vi "ADCP_Processed_Bytes_To_Data_Packet.vi"(8 "error in (no error)":errorcluster, 9 "Processed Packet":u8[](array[numeric])=[0, 0, 0, 0, 0, 0, 0, 0, 0], 10 "Data Packet In":T2, 11 "ADCP in":refnum<class "ADCP.lvclass">) -> (0 "error out":errorcluster, 2 "Data Packet Out":T2, 3 "ADCP out":refnum<class "ADCP.lvclass">)   [LabVIEW 2017, in "ADCP.lvclass"]
uses:
  ADCP.lvclass
  ADCP_Data_Packet_Transmit_Mode.ctl
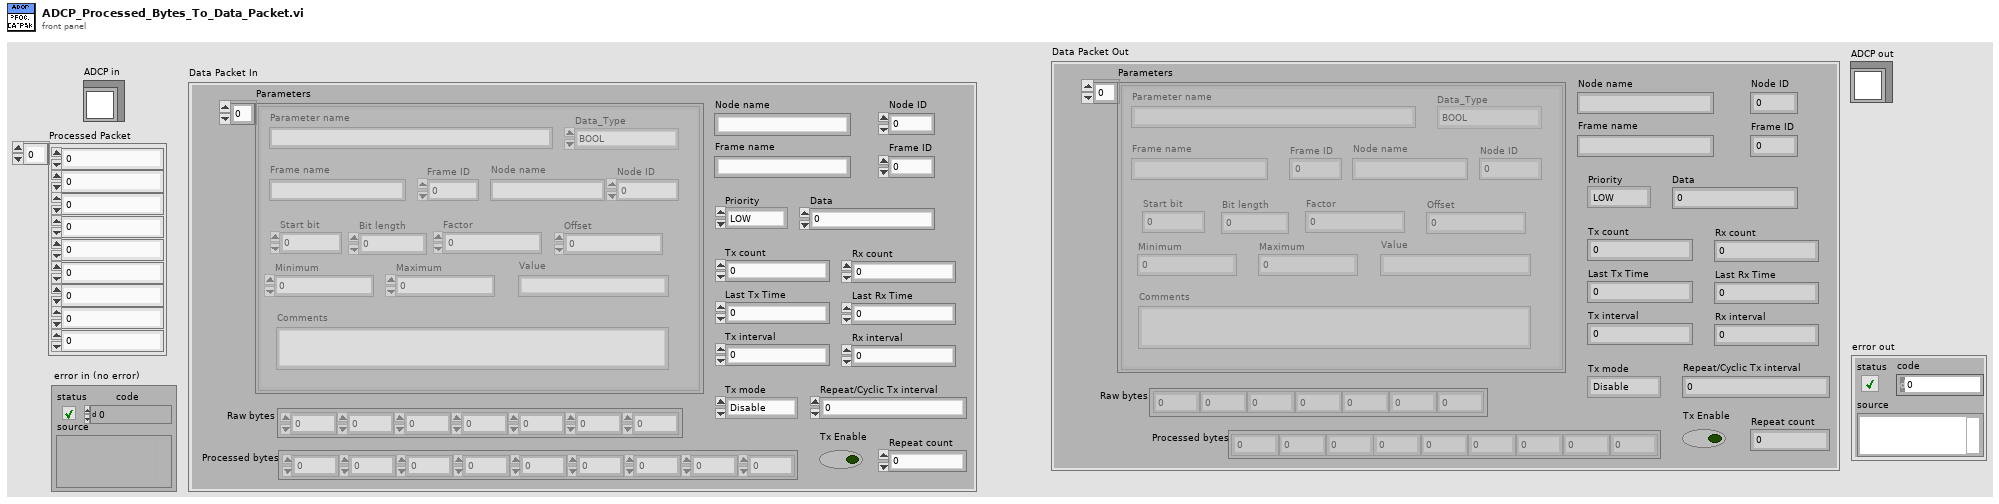
[diagram p1: front panel]
types:
  T1 = typedef "ADCP.lvclass/ADCP_Data_Packet_Transmit_Mode.ctl" = enum16{"Disable", "Single", "Cyclic", "Repeat"}
  T2 = cluster{"Parameters":cluster{"Parameter name":string, "Node name":string, "Node ID":u8, "Frame name":string, "Frame ID":u8, "Start bit":u32, "Bit length":u32, "Factor":dbl, "Offset":dbl, "Minimum":dbl, "Maximum":dbl, "Value":string, "Comments":string, "Data_Type":enum16{"BOOL", "UNSIGNED", "SIGNED", "FLOAT32", "ENUM"}}[], "Priority":enum16{"LOW", "HIGH"}, "Node name":string, "Node ID":u8, "Frame name":string, "Frame ID":u8, "Data":u32, "Raw bytes":u8[], "Processed bytes":u8[], "Tx count":i32, "Last Tx Time":u32, "Tx interval":u32, "Rx count":i32, "Last Rx Time":u32, "Rx interval":u32, "Tx Enable":bool, "Tx mode":T1, "Repeat/Cyclic Tx interval":u32, "Repeat count":u16}
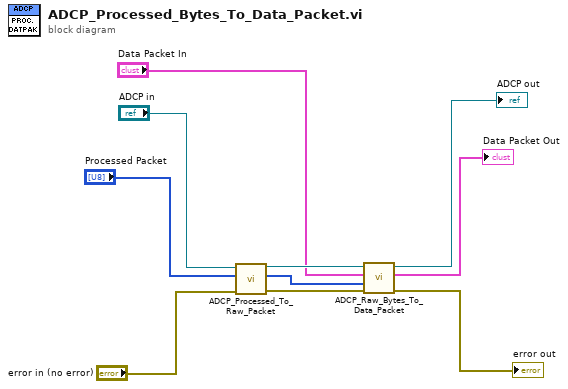
[diagram p0: block diagram]
diagram:
  n1 = call "ADCP_Processed_To_Raw_Packet.vi"("error in (no error)"="error in (no error)", "Processed Packet"="Processed Packet", "ADCP in"="ADCP in") -> ("error out"=w10:errorcluster, "Raw Packet"=w5:u8[], "ADCP out"=w9:refnum<class "ADCP.lvclass">)  [unwired: 6 in]
  n2 = call "ADCP_Raw_Bytes_To_Data_Packet.vi"("error in (no error)"=w10, "Raw Packet"=w5, "Data Packet In"="Data Packet In", "ADCP in"=w9) -> ("error out"=→"error out":errorcluster, "Data Packet Out"=→"Data Packet Out":T2, "ADCP out"=→"ADCP out":refnum<class "ADCP.lvclass">)  [unwired: 5 in]
